vi "CDM_0@6.vi"(8 "err in":errorcluster, 9 "Cpc":dbl, 10 "Pénalité":dbl, 11 "Qa":dbl) -> (0 "err out":errorcluster, 3 "CDM":dbl)   [LabVIEW 2010, in "lv_07.lvlib"]
doc: "Calcul du CDM annuel en cas de non stockage en fonction de de la pénalité encourue pour chaque défaillance (Pénalité), du coût d'une commande en urgence (Cpc). et de la consommation annuelle Qa"
uses:
  lv_07.lvlib
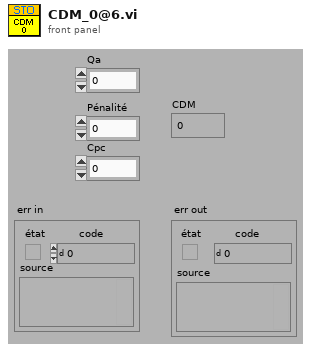
[diagram p1: front panel]
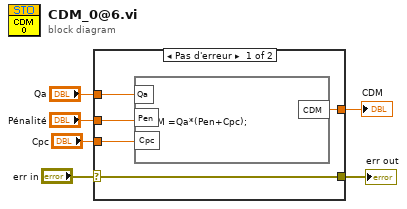
[diagram p0: block diagram]
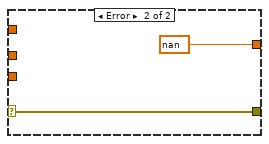
[diagram p2: hidden frame]
diagram:
  n1 = case shown="Pas d'erreur" "err in" {
    selector: "err in" -> [w7 w13]
    tunnel: [w7 w13] -> w5
    tunnel: "Qa" -> [w9 _]
    tunnel: "Pénalité" -> [w11 _]
    tunnel: "Cpc" -> [w10 _]
    tunnel: [w8 nan ("CDM")] -> w1
    frame No Error {
      n2 = formula code="CDM =Qa*(Pen+Cpc);"("Qa"=w9, "Pen"=w11, "Cpc"=w10) -> ("CDM"=w8:dbl)
    }
    frame Error {
    }
  }
  "err out" <- w5
  "CDM" <- w1
